vi "Periodic Tasks.vi"(0 "error in":errorcluster) -> ()   [LabVIEW 2018]
doc: "This VI runs in parallel to other tasks. It can contain as many user-defined periodic loops as you need. These can carry out PID or other sorts of timed response."
uses:
  <vilib>/Rock Robotics/WPI/Solenoid/WPI_SolenoidValue.ctl
  a5c3bee8-0f32-4d37-ac35-298c408eed11.vi
  ee49a8d8-d362-4c81-9a4d-ddfdb104c9cd.vi
  dsdata.vi
  instructions.vi
  constants.vi
  refnums.vi
  outputs.vi
  <vilib>/Rock Robotics/WPI/Solenoid/WPI_SolenoidSetEnum.vi
panel:
  out "Drive Sequencer":i32
  out "Subsystem Mode":path
  out "Driver_A":bool
  out "Time Since Latch (ms)":u32
  out "Subsystem Sequencer":i32
  out "Drive Mode":string
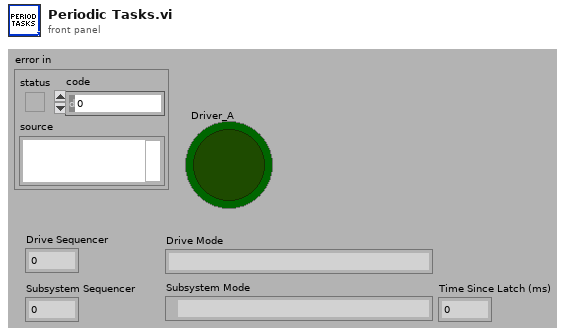
[diagram p1: front panel]
types:
  T1 = typedef "WPI_MotorControlDeviceRef.ctl" = cluster{"DeviceStatus":errorcluster, "Type":T2, "PWM":cluster{"PWM Channel":T3, "DeadBand":T4}, "CAN":cluster{"Device Number":u8, "SetOutput VI Ref":variant, "GetOutput VI Ref":variant, "Enable VI Ref":variant, "Disable VI Ref":variant, "Data":variant}, "Invert":bool, "DIO PWM":cluster{"PWM \"Enable\" Channel":T3, "DIOChannel":T5, "PWM Rate":dbl}}
  T2 = typedef "WPI_MotorControlType.ctl" = enum16{"PWM", "CAN", "DIO PWM"}
  T3 = typedef "FPGA_DIOPWMChannel.ctl" = enum8{"PWM 0", "PWM 1", "PWM 2", "PWM 3", "PWM 4", "PWM 5", "PWM 6", "PWM 7", "PWM 8", "PWM 9", "PWM MXP 0", "PWM MXP 1", "PWM MXP 2", "PWM MXP 3", "PWM MXP 4", "PWM MXP 5", "PWM MXP 6", "PWM MXP 7", "PWM MXP 8", "PWM MXP 9", "Invalid"}
  T4 = typedef "WPI_PWMDeadband.ctl" = cluster{"Name":string, "maxPositivePwm":i32, "minPositivePwm":i32, "centerPwm":i32, "maxNegativePwm":i32, "minNegativePwm":i32, "angularRange":u16}
  T5 = typedef "FPGA_DIOChannel.ctl" = enum8{"DIO 0", "DIO 1", "DIO 2", "DIO 3", "DIO 4", "DIO 5", "DIO 6", "DIO 7", "DIO 8", "DIO 9", "DIO MXP 0", "DIO MXP 1", "DIO MXP 2", "DIO MXP 3", "DIO MXP 4", "DIO MXP 5", "DIO MXP 6", "DIO MXP 7", "DIO MXP 8", "DIO MXP 9", "DIO MXP 10", "DIO MXP 11", "DIO MXP 12", "DIO MXP 13", "DIO MXP 14", "DIO MXP 15", "SPI Port CS1", "SPI Port CS2", "SPI Port CS3", "SPI Port MISO", "SPI Port MOSI", "Invalid"}
  T6 = typedef "WPI_SolenoidDevRef.ctl" = cluster{"DevStatus":errorcluster, "Pneumatics Control Module":u8, "Forward Solenoid Channel":T7, "Reverse Solenoid Channel":T7}
  T7 = typedef "WPI_SolenoidChannel.ctl" = enum8{"Solenoid 0", "Solenoid 1", "Solenoid 2", "Solenoid 3", "Solenoid 4", "Solenoid 5", "Solenoid 6", "Solenoid 7", "Invalid"}
  T8 = typedef "WPI_DriverStationRobotMode2.ctl" = enum16{"Autonomous Disabled", "Autonomous Enabled", "Teleop Disabled", "Teleop Enabled", "Disconnected", "Finish", "Test Disabled", "Test Enabled", "Emergency Stopped"}
  T9 = typedef "WPI_SolenoidValue.ctl" = enum16{"Off", "On", "Forward", "Reverse"}
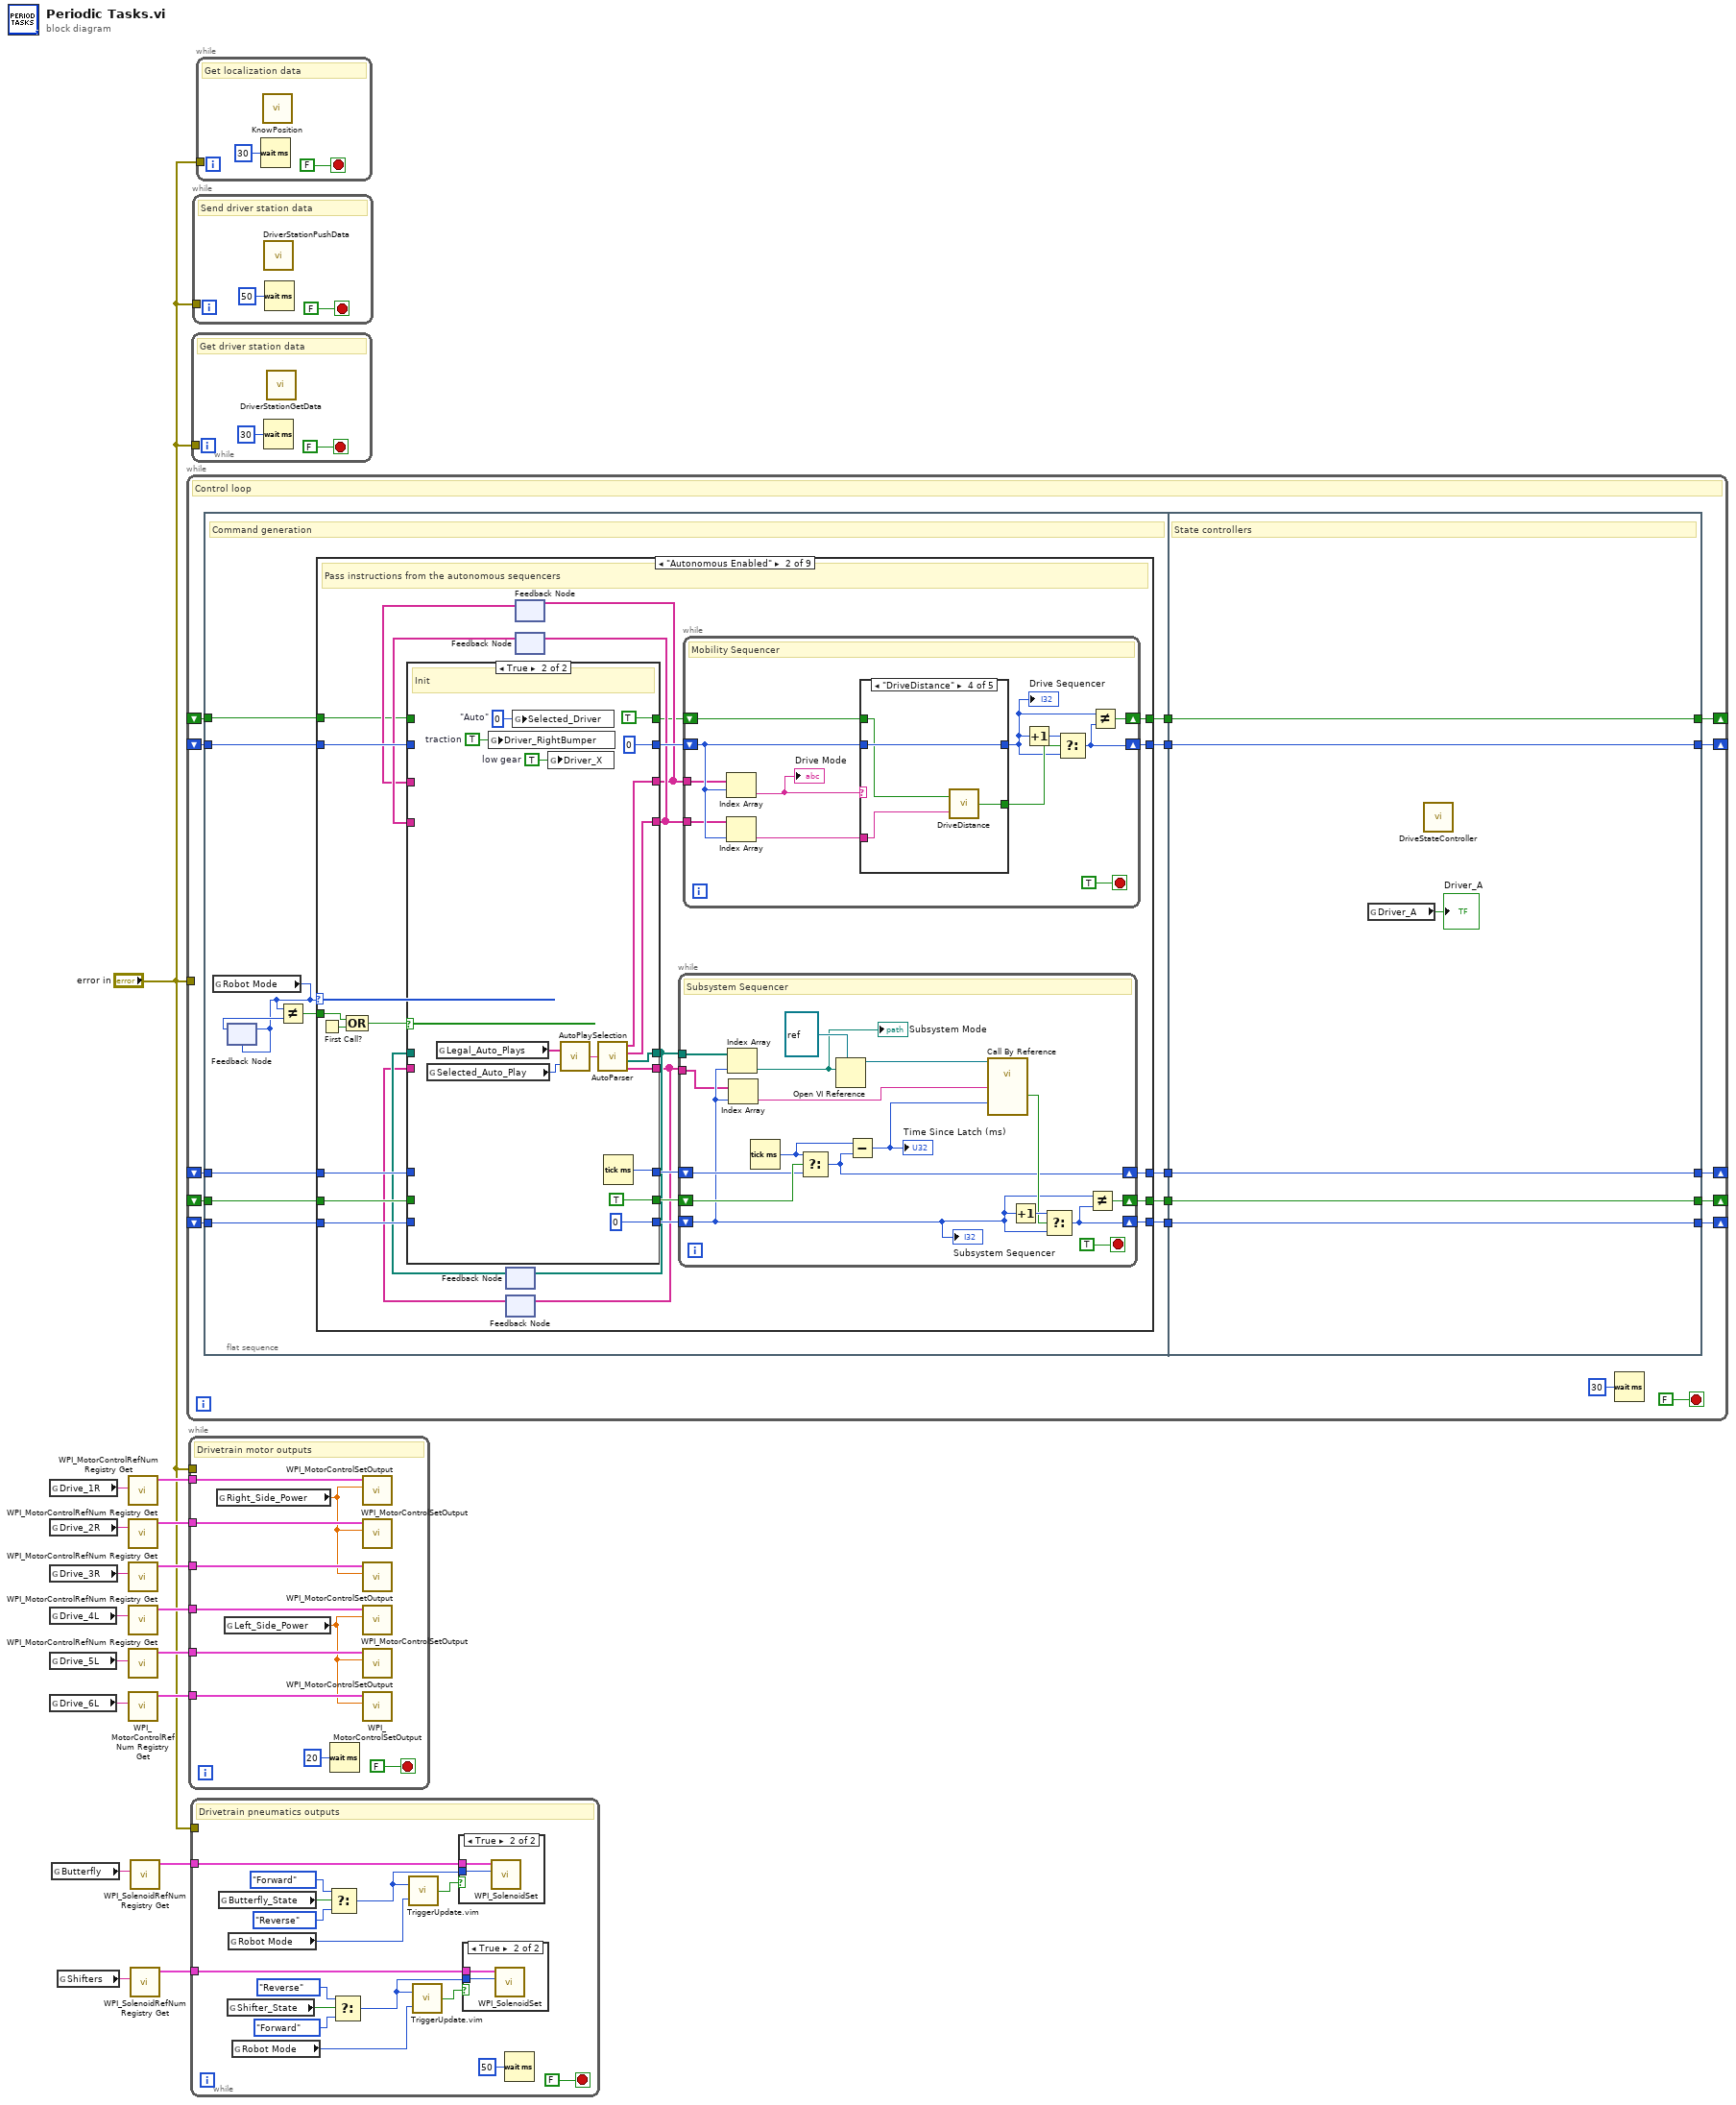
[diagram p0: block diagram]
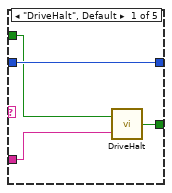
[diagram p5: hidden frame]
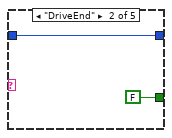
[diagram p6: hidden frame]
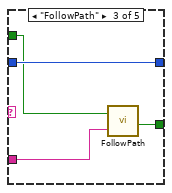
[diagram p7: hidden frame]
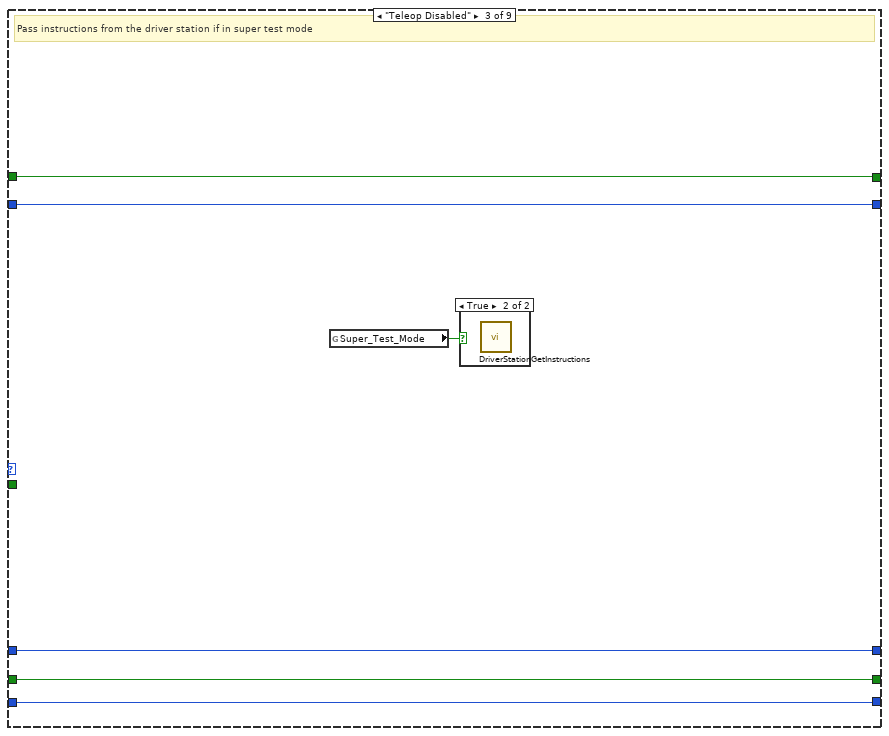
[diagram p10: hidden frame]
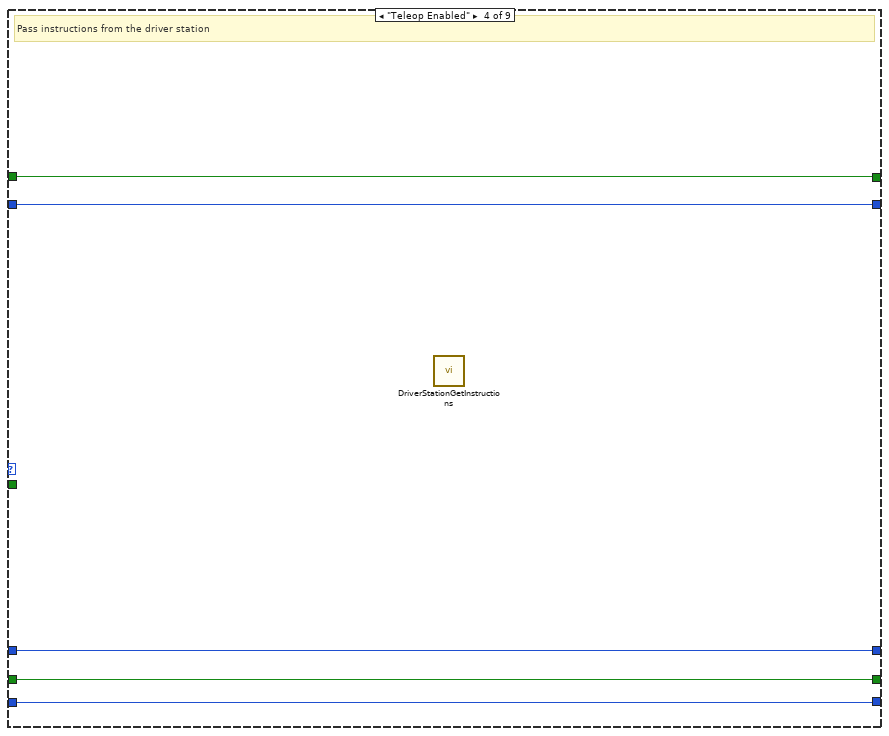
[diagram p12: hidden frame]
diagram:
  n1 = global read "refnums.vi" "Drive_1R"() -> (w11:string)
  n2 = global read "refnums.vi" "Drive_2R"() -> (w10:string)
  n3 = global read "refnums.vi" "Drive_3R"() -> (w9:string)
  n4 = global read "refnums.vi" "Drive_4L"() -> (w8:string)
  n5 = global read "refnums.vi" "Drive_5L"() -> (w7:string)
  n6 = global read "refnums.vi" "Drive_6L"() -> (w6:string)
  n7 = global read "refnums.vi" "Butterfly"() -> (w4:string)
  n8 = global read "refnums.vi" "Shifters"() -> (w3:string)
  n9 = call <vilib>:"WPI_MotorControlRefNum Registry Get.vi"("refnum name"=w11) -> ("MotorControlDevRef"=w17:T1)  [unwired: 9 in, 1 out]
  n10 = call <vilib>:"WPI_MotorControlRefNum Registry Get.vi"("refnum name"=w10) -> ("MotorControlDevRef"=w16:T1)  [unwired: 9 in, 1 out]
  n11 = call <vilib>:"WPI_MotorControlRefNum Registry Get.vi"("refnum name"=w9) -> ("MotorControlDevRef"=w15:T1)  [unwired: 9 in, 1 out]
  n12 = call <vilib>:"WPI_MotorControlRefNum Registry Get.vi"("refnum name"=w8) -> ("MotorControlDevRef"=w14:T1)  [unwired: 9 in, 1 out]
  n13 = call <vilib>:"WPI_MotorControlRefNum Registry Get.vi"("refnum name"=w7) -> ("MotorControlDevRef"=w13:T1)  [unwired: 9 in, 1 out]
  n14 = call <vilib>:"WPI_MotorControlRefNum Registry Get.vi"("refnum name"=w6) -> ("MotorControlDevRef"=w12:T1)  [unwired: 9 in, 1 out]
  n15 = call <vilib>:"WPI_SolenoidRefNum Registry Get.vi"("refnum name"=w4) -> ("SolenoidDevRef"=w5:T6)  [unwired: 9 in, 1 out]
  n16 = call <vilib>:"WPI_SolenoidRefNum Registry Get.vi"("refnum name"=w3) -> ("SolenoidDevRef"=w2:T6)  [unwired: 9 in, 1 out]
  n17 = while {
    tunnel: "error in" -> [_]
    shift-right: [w24] -> _
    shift-left: _ -> [w30]
    shift-right: [w25] -> _
    shift-left: _ -> [w31]
    shift-right: [w26] -> _
    shift-left: _ -> [w32]
    shift-right: [w22] -> _
    shift-left: _ -> [w21]
    shift-right: [w19] -> _
    shift-left: _ -> [w18]
    stop <- FALSE stop-if-true
    # "Control loop"
    n18 = flat-sequence {
      tunnel: w32 -> [w44]
      tunnel: w31 -> [w43]
      tunnel: w30 -> [w42]
      tunnel: [w47] -> w29
      tunnel: [w46] -> w28
      tunnel: [w45] -> w27
      tunnel: [w39] -> w23
      tunnel: w21 -> [w38]
      tunnel: [w37] -> w20
      tunnel: w18 -> [w36]
      tunnel: w29 -> [w188]
      tunnel: w28 -> [w187]
      tunnel: w27 -> [w186]
      tunnel: [w188] -> w26
      tunnel: [w187] -> w25
      tunnel: [w186] -> w24
      tunnel: w23 -> [w185]
      tunnel: [w185] -> w22
      tunnel: [w184] -> w19
      tunnel: w20 -> [w184]
      frame #0 {
        # "Command generation"
        n19 = global read "dsdata.vi" "Robot Mode"() -> (w35:T8)
        n20 = feedback-in #1(w35) -> ()
        n21 = feedback #1(w35) -> (w41:T8)
        n22 = Not Equal?(x=w35, y=w41) -> (x != y?=w40:bool)
        n23 = case shown="\"Autonomous Enabled\"" w35 {
          tunnel: w44 -> [w52 w75 w150 w155 w160 w165 w170 w175 w180]
          tunnel: w43 -> [w51 w73 w149 w154 w159 w164 w169 w174 w179]
          tunnel: w42 -> [w50 w72 w148 w153 w158 w163 w168 w173 w178]
          tunnel: [w52 w78 w150 w155 w160 w165 w170 w175 w180] -> w47
          tunnel: [w51 w77 w149 w154 w159 w164 w169 w174 w179] -> w46
          tunnel: [w50 w76 w148 w153 w158 w163 w168 w173 w178] -> w45
          tunnel: w40 -> [_ w67 _ _ _ _ _ _ _]
          tunnel: [w49 w61 w151 w156 w161 w166 w171 w176 w181] -> w39
          tunnel: w38 -> [w49 w60 w151 w156 w161 w166 w171 w176 w181]
          tunnel: [w48 w54 w152 w157 w162 w167 w172 w177 w182] -> w37
          tunnel: w36 -> [w48 w53 w152 w157 w162 w167 w172 w177 w182]
          frame "Autonomous Disabled", Default {
          }
          frame "Autonomous Enabled" {
            # "Pass instructions from the autonomous sequencers"
            n24 = First Call?() -> (First Call?: T/F=w68:bool)
            n25 = Compound Arithmetic op=OR(w67, w68) -> (w69:bool)
            n26 = feedback #2() -> (w64:path[])  [unwired: 1 in]
            n27 = feedback #3() -> (w63:string[])  [unwired: 1 in]
            n28 = feedback #4() -> (w56:string[])  [unwired: 1 in]
            n29 = feedback #5() -> (w57:string[])  [unwired: 1 in]
            n30 = case shown="True" w69 {
              tunnel: w72 -> [w112 _]
              tunnel: w73 -> [w113 _]
              tunnel: w75 -> [w114 _]
              tunnel: [w114 w129] -> w74
              tunnel: [w113 TRUE ("Advance Trigger")] -> w71
              tunnel: [w112 0] -> w70
              tunnel: [w111 w122] -> w66
              tunnel: [w110 w126] -> w65
              tunnel: w64 -> [w111 _]
              tunnel: w63 -> [w110 _]
              tunnel: [w109 0] -> w62
              tunnel: w60 -> [w109 _]
              tunnel: [w108 w124] -> w59
              tunnel: [w107 w123] -> w58
              tunnel: w57 -> [w108 _]
              tunnel: w56 -> [w107 _]
              tunnel: [w106 TRUE] -> w55
              tunnel: w53 -> [w106 _]
              frame False {
                # "Pass"
              }
              frame True {
                w118 = TRUE  # low gear
                w119 = TRUE  # traction
                w120 = 0  # "Auto"
                # "Init"
                n31 = global read "dsdata.vi" "Selected_Auto_Play"() -> (w117:u16)
                n32 = global read "constants.vi" "Legal_Auto_Plays"() -> (w116:string[])
                n33 = global write "instructions.vi" "Driver_RightBumper"(w119) -> ()
                n34 = global write "instructions.vi" "Selected_Driver"(w120) -> ()
                n35 = global write "instructions.vi" "Driver_X"(w118) -> ()
                n36 = call "AutoPlaySelection.vi"("Selected Auto Play"=w117, "Auto Plays"=w116) -> ("Autonomous Commands"=w115:string)
                n37 = call "AutoParser.vi"("Auto Play"=w115) -> ("Drive Mode Strings"=w123:string[], "Drive Command Strings"=w124:string[], "Subsystem VI References"=w122:path[], "Subsystem Command Strings"=w126:string[])
                n38 = Tick Count (ms)() -> (millisecond timer value=w129:u32)
              }
            }
            n39 = feedback-in #2(w66) -> ()
            n40 = feedback-in #3(w65) -> ()
            n41 = feedback-in #4(w58) -> ()
            n42 = feedback-in #5(w59) -> ()
            n43 = while {
              tunnel: w66 -> [w134]
              shift-right: [w142] -> w76
              shift-left: w70 -> [w132]
              shift-right: [w141] -> w77
              shift-left: w71 -> [w140]
              shift-right: [w138] -> w78
              shift-left: w74 -> [w139]
              tunnel: w65 -> [w131]
              stop <- TRUE stop-if-true
              # "Subsystem Sequencer"
              n44 = Index Array(array=w134, index=w132) -> (element=w133:path)
              "Subsystem Mode" <- w133
              n45 = Index Array(array=w131, index=w132) -> (element=w130:string)
              n46 = Tick Count (ms)() -> (millisecond timer value=w137:u32)
              n47 = Select(t=w137, s=w140, f=w139) -> (s? t:f=w138:u32)
              n48 = Open VI Reference(type specifier VI Refnum (for type only)=refnum<vi> refnum, vi path=w133) -> (vi reference=w136:refnum<vi>)  [unwired: 4 in, 1 out]
              n49 = Subtract(x=w137, y=w138) -> (x-y=w135:u32)
              "Time Since Latch (ms)" <- w135
              n50 = call-by-ref "?"(reference=w136, "Time Since Latch"=w135, "Instruction String"=w130) -> ("Advance Trigger"=w143:bool)  [unwired: 1 in, 2 out]
              n51 = Increment(x=w132) -> (x+1=w145:i32)
              n52 = Select(t=w145, s=w143, f=w132) -> (s? t:f=w142:i32)
              n53 = Not Equal?(x=w132, y=w142) -> (x != y?=w141:bool)
              "Subsystem Sequencer" <- w132
            }
            n54 = while {
              shift-right: [w82] -> w61
              shift-left: w62 -> [w88]
              tunnel: w58 -> [w87]
              tunnel: w59 -> [w86]
              shift-right: [w81] -> w54
              shift-left: w55 -> [w80]
              stop <- TRUE stop-if-true
              # "Mobility Sequencer"
              n55 = Index Array(array=w87, index=w88) -> (element=w85:string)
              "Drive Mode" <- w85
              n56 = Index Array(array=w86, index=w88) -> (element=w84:string)
              n57 = case shown="\"DriveDistance\"" w85 {
                tunnel: w88 -> [w94 w96 w100 w104 w105]
                tunnel: [w94 w96 w100 w104 w105] -> w79
                tunnel: w84 -> [w91 _ w97 w102 _]
                tunnel: [w93 FALSE ("Increment") w99 w101 _] -> w83
                tunnel: w80 -> [w92 _ w98 w103 _]
                frame "DriveHalt", Default {
                  n58 = call "DriveHalt.vi"("Parameter String"=w91, "Reinit"=w92) -> ("Increment"=w93:bool)
                }
                frame "DriveEnd" {
                }
                frame "FollowPath" {
                  n59 = call "FollowPath.vi"("Parameter String"=w97, "Reinit"=w98) -> ("Increment"=w99:bool)
                }
                frame "DriveDistance" {
                  n60 = call "DriveDistance.vi"("Parameter String"=w102, "Reinit"=w103) -> ("Increment"=w101:bool)
                }
                frame "RotateAngle" {
                }
              }
              "Drive Sequencer" <- w79
              n61 = Increment(x=w79) -> (x+1=w89:i32)
              n62 = Select(t=w89, s=w83, f=w79) -> (s? t:f=w82:i32)
              n63 = Not Equal?(x=w79, y=w82) -> (x != y?=w81:bool)
            }
          }
          frame "Teleop Disabled" {
            # "Pass instructions from the driver station if in super test mode"
            n64 = global read "dsdata.vi" "Super_Test_Mode"() -> (w147:bool)
            n65 = case shown="True" w147 {
              frame False {
              }
              frame True {
                n66 = call "DriverStationGetInstructions.vi"() -> ()  [unwired: 12 in]
              }
            }
          }
          frame "Teleop Enabled" {
            # "Pass instructions from the driver station"
            n67 = call "DriverStationGetInstructions.vi"() -> ()  [unwired: 12 in]
          }
          frame "Finish" {
          }
          frame "Test Disabled" {
          }
          frame "Test Enabled" {
          }
          frame "Disconnected" {
          }
          frame "Emergency Stopped" {
          }
        }
      }
      frame #1 {
        # "State controllers"
        n68 = global read "instructions.vi" "Driver_A"() -> (→"Driver_A":bool)
        n69 = call "DriveStateController.vi"() -> ()  [unwired: 1 in]
      }
    }
    n70 = Wait (ms)(milliseconds to wait=u32 30) -> ()  [unwired: 1 out]
  }
  n71 = while {
    tunnel: "error in" -> [_]
    tunnel: w17 -> [w196]
    tunnel: w16 -> [w195]
    tunnel: w15 -> [w194]
    tunnel: w14 -> [w193]
    tunnel: w13 -> [w192]
    tunnel: w12 -> [w191]
    stop <- FALSE stop-if-true
    # "Drivetrain motor outputs"
    n72 = global read "outputs.vi" "Right_Side_Power"() -> (w190:dbl)
    n73 = global read "outputs.vi" "Left_Side_Power"() -> (w189:dbl)
    n74 = Wait (ms)(milliseconds to wait=u32 20) -> ()  [unwired: 1 out]
    n75 = call <vilib>:"WPI_MotorControlSetOutput.vi"("Output"=w190, "MotorControlDevRef"=w196) -> ()  [unwired: 7 in, 3 out]
    n76 = call <vilib>:"WPI_MotorControlSetOutput.vi"("Output"=w190, "MotorControlDevRef"=w195) -> ()  [unwired: 7 in, 3 out]
    n77 = call <vilib>:"WPI_MotorControlSetOutput.vi"("Output"=w190, "MotorControlDevRef"=w194) -> ()  [unwired: 7 in, 3 out]
    n78 = call <vilib>:"WPI_MotorControlSetOutput.vi"("Output"=w189, "MotorControlDevRef"=w193) -> ()  [unwired: 7 in, 3 out]
    n79 = call <vilib>:"WPI_MotorControlSetOutput.vi"("Output"=w189, "MotorControlDevRef"=w192) -> ()  [unwired: 7 in, 3 out]
    n80 = call <vilib>:"WPI_MotorControlSetOutput.vi"("Output"=w189, "MotorControlDevRef"=w191) -> ()  [unwired: 7 in, 3 out]
  }
  n81 = while {
    tunnel: "error in" -> [_]
    tunnel: w5 -> [w209]
    tunnel: w2 -> [w200]
    stop <- FALSE stop-if-true
    # "Drivetrain pneumatics outputs"
    n82 = global read "outputs.vi" "Butterfly_State"() -> (w207:bool)
    n83 = global read "outputs.vi" "Shifter_State"() -> (w201:bool)
    n84 = global read "dsdata.vi" "Robot Mode"() -> (w208:T8)
    n85 = global read "dsdata.vi" "Robot Mode"() -> (w202:T8)
    n86 = Select(t=WPI_SolenoidValue."Forward" ("Value"), s=w207, f=WPI_SolenoidValue."Reverse" ("Value")) -> (s? t:f=w211:T9)
    n87 = Select(t=WPI_SolenoidValue."Reverse" ("Value"), s=w201, f=WPI_SolenoidValue."Forward" ("Value")) -> (s? t:f=w204:T9)
    n88 = call "TriggerUpdate.vim"("Robot Mode"=w208, "Trigger"=w211) -> ("Update"=w210:bool)
    n89 = call "TriggerUpdate.vim"("Robot Mode"=w202, "Trigger"=w204) -> ("Update"=w203:bool)
    n90 = case shown="True" w210 {
      tunnel: w211 -> [_ w218]
      tunnel: w209 -> [_ w217]
      frame False {
      }
      frame True {
        n91 = call-poly <vilib>:"WPI_SolenoidSet.vi"("Value"=w218, "SolenoidDevRef"=w217) -> ()  [unwired: 8 in, 2 out]
      }
    }
    n92 = case shown="True" w203 {
      tunnel: w204 -> [_ w216]
      tunnel: w200 -> [_ w215]
      frame False {
      }
      frame True {
        n93 = call-poly <vilib>:"WPI_SolenoidSet.vi"("Value"=w216, "SolenoidDevRef"=w215) -> ()  [unwired: 8 in, 2 out]
      }
    }
    n94 = Wait (ms)(milliseconds to wait=u32 50) -> ()  [unwired: 1 out]
  }
  n95 = while {
    tunnel: "error in" -> [_]
    stop <- FALSE stop-if-true
    # "Get driver station data"
    n96 = Wait (ms)(milliseconds to wait=u32 30) -> ()  [unwired: 1 out]
    n97 = call "DriverStationGetData.vi"() -> ()  [unwired: 1 in]
  }
  n98 = while {
    tunnel: "error in" -> [_]
    stop <- FALSE stop-if-true
    # "Send driver station data"
    n99 = call "DriverStationPushData.vi"() -> ()  [unwired: 12 in]
    n100 = Wait (ms)(milliseconds to wait=u32 50) -> ()  [unwired: 1 out]
  }
  n101 = while {
    tunnel: "error in" -> [_]
    stop <- FALSE stop-if-true
    # "Get localization data"
    n102 = Wait (ms)(milliseconds to wait=u32 30) -> ()  [unwired: 1 out]
    n103 = call "KnowPosition.vi"() -> ()  [unwired: 1 in]
  }
